vi "_builtins_rect_to_relative_move.vi"(10 "End Rects out":T1[](array[typedef]), 11 "Start Rects in":T1[](array[typedef])) -> (3 "Relative Move":T2[](array[typedef]))   [LabVIEW 2019, in "Script.lvlib"]
doc: "Resolves the relative move from the start and end rectangle bounds.\n\nCreated by: Ryan Pacini"
uses:
  Script.lvlib
  <vilib>/Utility/miscctls.llb/LVRectTypeDef.ctl
  <vilib>/Utility/miscctls.llb/LVPositionTypeDef.ctl
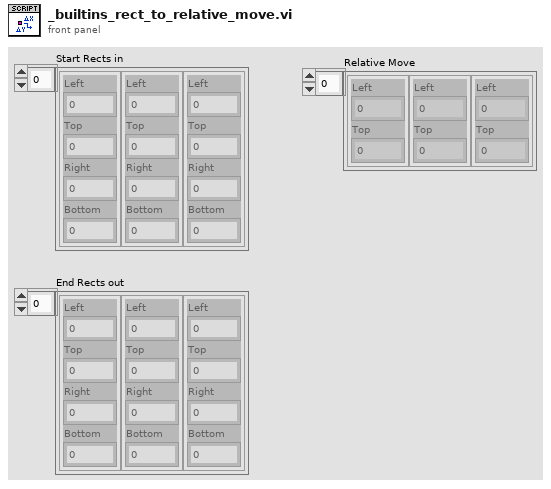
[diagram p1: front panel]
types:
  T1 = typedef "LVRectTypeDef.ctl" = cluster{"Left":i16, "Top":i16, "Right":i16, "Bottom":i16}
  T2 = typedef "LVPositionTypeDef.ctl" = cluster{"Left":i32, "Top":i32}
  T3 = cluster{"Left":i32, "Top":i32, "Right":i32, "Bottom":i32}
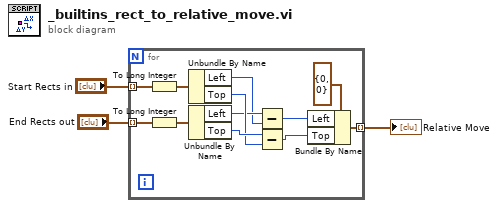
[diagram p0: block diagram]
diagram:
  n1 = for {
    tunnel: "Start Rects in" -> [w15] mode=indexing
    tunnel: "End Rects out" -> [w14] mode=indexing
    tunnel: [w4] -> w2 mode=indexing
    n2 = To Long Integer(number=w15) -> (32bit integer=w6:T3)
    n3 = To Long Integer(number=w14) -> (32bit integer=w5:T3)
    n4 = Unbundle By Name(w6) -> ("Left"=w10:i32, "Top"=w12:i32)
    n5 = Unbundle By Name(w5) -> ("Left"=w11:i32, "Top"=w13:i32)
    n6 = Subtract(x=w11, y=w10) -> (x-y=w8:i32)
    n7 = Subtract(x=w13, y=w12) -> (x-y=w7:i32)
    n8 = Bundle By Name(cluster=T2 {"Left"=0, "Top"=0} ("Position"), "Left"=w8, "Top"=w7) -> (w4:T2)
  }
  "Relative Move" <- w2
